vi "TestData.vi"(6 "Reading No.":u32, 7 "Action":enum16{"Reset", "Write Element", "Read Array"}(ring), 8 "Test No.":u32, 9 "Array No.":u32, 10 "Data IN":dbl format="%.2f", 11 "Data IN":cluster{dbl[], dbl[], dbl[], dbl[], dbl[]}[](array[cluster])) -> (2 "Array OUT":dbl[](array[numeric]), 3 "Data OUT":cluster{dbl[], dbl[], dbl[], dbl[], dbl[]}[](array[cluster]))   [LabVIEW 2019]
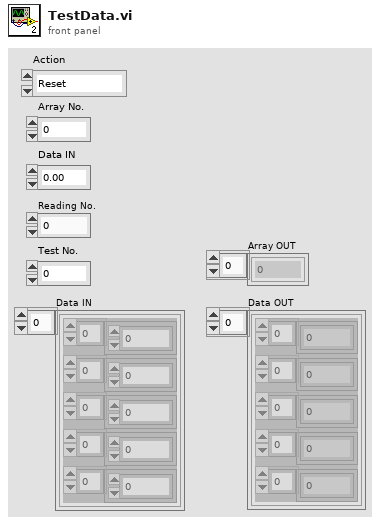
[diagram p1: front panel]
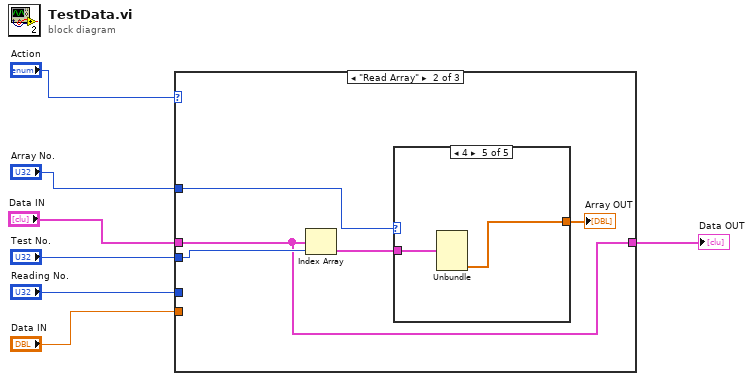
[diagram p0: block diagram]
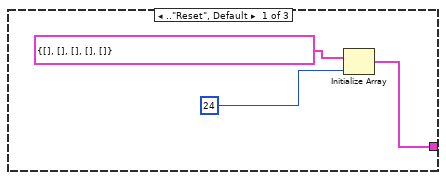
[diagram p2: hidden frame]
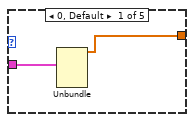
[diagram p3: hidden frame]
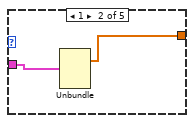
[diagram p4: hidden frame]
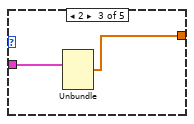
[diagram p5: hidden frame]
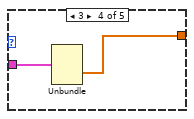
[diagram p6: hidden frame]
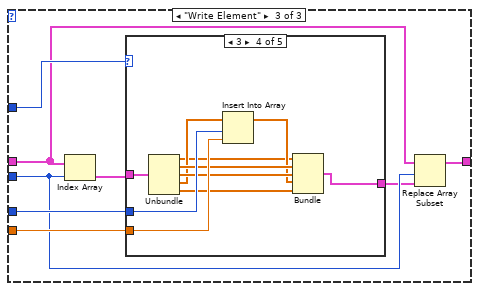
[diagram p7: hidden frame]
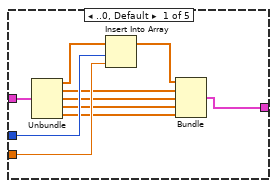
[diagram p8: hidden frame]
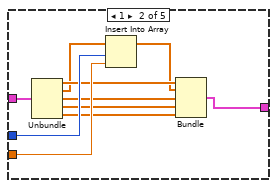
[diagram p9: hidden frame]
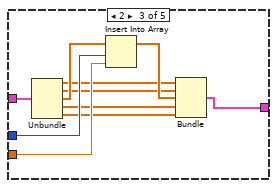
[diagram p10: hidden frame]
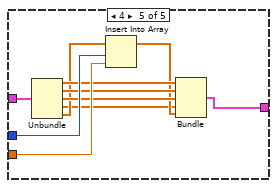
[diagram p11: hidden frame]
diagram:
  n1 = case shown="\"Read Array\"" "Action" {
    tunnel: "Test No." -> [_ w14 w28]
    tunnel: "Data IN" -> [_ _ w32]
    tunnel: "Array No." -> [_ w13 w33]
    tunnel: [w9 w11 w31] -> w2
    tunnel: "Data IN" -> [_ w11 w26]
    tunnel: "Reading No." -> [_ _ w29]
    frame .."Reset", Default {
      n2 = Initialize Array(cluster{dbl[], dbl[], dbl[], dbl[], dbl[]} {[], [], [], [], []}, 24 ("dimension size")) -> (w9:cluster{dbl[], dbl[], dbl[], dbl[], dbl[]}[])
    }
    frame "Read Array" {
      n3 = Index Array(array=w11, index=w14) -> (element=w15:cluster{dbl[], dbl[], dbl[], dbl[], dbl[]})
      n4 = case shown="4" w13 {
        tunnel: w15 -> [w17 w19 w21 w23 w25]
        tunnel: [w16 w18 w20 w22 w24] -> w12
        frame 0, Default {
          n5 = Unbundle(w17) -> (w16:dbl[])  [unwired: 4 out]
        }
        frame 1 {
          n6 = Unbundle(w19) -> (w18:dbl[])  [unwired: 4 out]
        }
        frame 2 {
          n7 = Unbundle(w21) -> (w20:dbl[])  [unwired: 4 out]
        }
        frame 3 {
          n8 = Unbundle(w23) -> (w22:dbl[])  [unwired: 4 out]
        }
        frame 4 {
          n9 = Unbundle(w25) -> (w24:dbl[])  [unwired: 4 out]
        }
      }
      "Array OUT" <- w12
    }
    frame "Write Element" {
      n10 = Index Array(array=w26, index=w28) -> (element=w30:cluster{dbl[], dbl[], dbl[], dbl[], dbl[]})
      n11 = case shown="3" w33 {
        tunnel: w32 -> [w40 w51 w61 w71 w81]
        tunnel: w30 -> [w43 w53 w63 w73 w83]
        tunnel: w29 -> [w41 w52 w62 w72 w82]
        tunnel: [w34 w47 w58 w67 w78] -> w27
        frame ..0, Default {
          n12 = Unbundle(w43) -> (w42:dbl[], w39:dbl[], w38:dbl[], w37:dbl[], w36:dbl[])
          n13 = Insert Into Array(array=w42, index=w41, new element=w40) -> (w35:dbl[])
          n14 = Bundle(w35, w39, w38, w37, w36) -> (w34:cluster{dbl[], dbl[], dbl[], dbl[], dbl[]})  [unwired: 1 in]
        }
        frame 1 {
          n15 = Unbundle(w53) -> (w46:dbl[], w45:dbl[], w50:dbl[], w49:dbl[], w48:dbl[])
          n16 = Insert Into Array(array=w45, index=w52, new element=w51) -> (w44:dbl[])
          n17 = Bundle(w46, w44, w50, w49, w48) -> (w47:cluster{dbl[], dbl[], dbl[], dbl[], dbl[]})  [unwired: 1 in]
        }
        frame 2 {
          n18 = Unbundle(w63) -> (w55:dbl[], w54:dbl[], w57:dbl[], w60:dbl[], w59:dbl[])
          n19 = Insert Into Array(array=w57, index=w62, new element=w61) -> (w56:dbl[])
          n20 = Bundle(w55, w54, w56, w60, w59) -> (w58:cluster{dbl[], dbl[], dbl[], dbl[], dbl[]})  [unwired: 1 in]
        }
        frame 3 {
          n21 = Unbundle(w73) -> (w64:dbl[], w70:dbl[], w69:dbl[], w66:dbl[], w68:dbl[])
          n22 = Insert Into Array(array=w66, index=w72, new element=w71) -> (w65:dbl[])
          n23 = Bundle(w64, w70, w69, w65, w68) -> (w67:cluster{dbl[], dbl[], dbl[], dbl[], dbl[]})  [unwired: 1 in]
        }
        frame 4 {
          n24 = Unbundle(w83) -> (w77:dbl[], w80:dbl[], w79:dbl[], w74:dbl[], w76:dbl[])
          n25 = Insert Into Array(array=w76, index=w82, new element=w81) -> (w75:dbl[])
          n26 = Bundle(w77, w80, w79, w74, w75) -> (w78:cluster{dbl[], dbl[], dbl[], dbl[], dbl[]})  [unwired: 1 in]
        }
      }
      n27 = Replace Array Subset(array=w26, new element=w27, index=w28) -> (w31:cluster{dbl[], dbl[], dbl[], dbl[], dbl[]}[])
    }
  }
  "Data OUT" <- w2
